vi "StateActuators.vi"(0 "Master State":enum16{"Normal"}(ring)) -> ()   [LabVIEW 2020]
uses:
  outputs.vi
  dscommands.vi
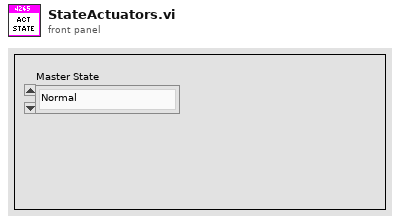
[diagram p1: front panel]
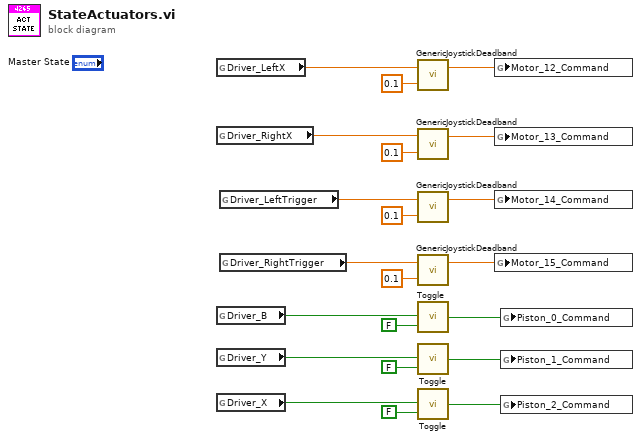
[diagram p0: block diagram]
diagram:
  n1 = global read "dscommands.vi" "Driver_LeftX"() -> (w21:dbl)
  n2 = global read "dscommands.vi" "Driver_RightX"() -> (w3:dbl)
  n3 = global read "dscommands.vi" "Driver_B"() -> (w14:bool)
  n4 = global read "dscommands.vi" "Driver_Y"() -> (w11:bool)
  n5 = global read "dscommands.vi" "Driver_X"() -> (w8:bool)
  n6 = global read "dscommands.vi" "Driver_LeftTrigger"() -> (w16:dbl)
  n7 = global read "dscommands.vi" "Driver_RightTrigger"() -> (w15:dbl)
  n8 = call "GenericJoystickDeadband.vi"("Deadband"=0.1, "Raw Joystick Value"=w21) -> ("Scaled Joystick Value"=w19:dbl)  [unwired: 1 in]
  n9 = call "GenericJoystickDeadband.vi"("Deadband"=0.1, "Raw Joystick Value"=w3) -> ("Scaled Joystick Value"=w4:dbl)  [unwired: 1 in]
  n10 = call "GenericJoystickDeadband.vi"("Deadband"=0.1, "Raw Joystick Value"=w16) -> ("Scaled Joystick Value"=w2:dbl)  [unwired: 1 in]
  n11 = call "GenericJoystickDeadband.vi"("Deadband"=0.1, "Raw Joystick Value"=w15) -> ("Scaled Joystick Value"=w1:dbl)  [unwired: 1 in]
  n12 = call "Toggle.vi"("Initial State"=FALSE, "Trigger"=w14) -> ("New State"=w13:bool)
  n13 = call "Toggle.vi"("Initial State"=FALSE, "Trigger"=w11) -> ("New State"=w10:bool)
  n14 = call "Toggle.vi"("Initial State"=FALSE, "Trigger"=w8) -> ("New State"=w7:bool)
  n15 = global write "outputs.vi" "Motor_12_Command"(w19) -> ()
  n16 = global write "outputs.vi" "Motor_13_Command"(w4) -> ()
  n17 = global write "outputs.vi" "Motor_14_Command"(w2) -> ()
  n18 = global write "outputs.vi" "Motor_15_Command"(w1) -> ()
  n19 = global write "outputs.vi" "Piston_0_Command"(w13) -> ()
  n20 = global write "outputs.vi" "Piston_1_Command"(w10) -> ()
  n21 = global write "outputs.vi" "Piston_2_Command"(w7) -> ()
